vi "Untitled 31 (SubVI).vi"(4 "Vneg":dbl, 5 "Cpos":dbl, 6 "TF output":dbl, 7 "Cneg":dbl, 11 "Vpos":dbl) -> (3 "output":dbl)   [LabVIEW 2021]
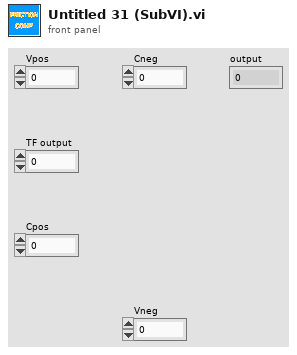
[diagram p1: front panel]
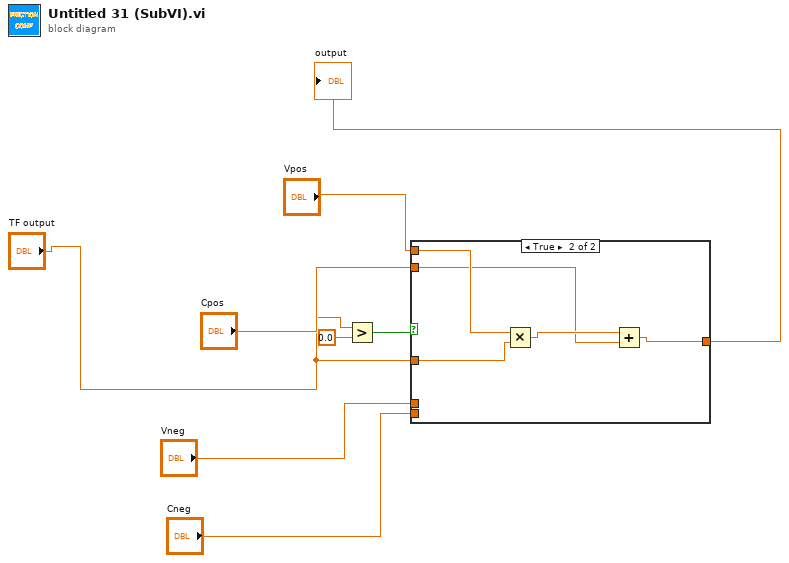
[diagram p0: block diagram]
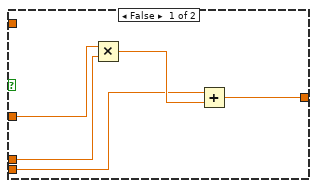
[diagram p2: hidden frame]
diagram:
  n1 = Greater?(x="TF output", y=0.0) -> (0:w2:bool)
  n2 = case shown="True" w2 {
    tunnel: [w9 w14] -> w1
    tunnel: "Vpos" -> [_ w18]
    tunnel: "TF output" -> [w10 w17]
    tunnel: "Cpos" -> [_ w15]
    tunnel: "Cneg" -> [w12 _]
    tunnel: "Vneg" -> [w11 _]
    frame False {
      n3 = Multiply ("Multiply 2")(x=w10, y=w11) -> (x*y=w13:dbl)
      n4 = Add ("Add 2")(x=w12, y=w13) -> (x+y=w9:dbl)
    }
    frame True {
      n5 = Multiply(x=w18, y=w17) -> (x*y=w16:dbl)
      n6 = Add(x=w16, y=w15) -> (x+y=w14:dbl)
    }
  }
  "output" <- w1
